vi "get RawTest filename.vi"(10 "Device Name":string, 11 "Wafer Name":string) -> (0 "current time":timestamp, 3 "FileName":string)   [LabVIEW 2012]
uses:
  <vilib>/Utility/miscctls.llb/LVDateTimeRec.ctl
panel:
  out "date/time string":string
  out "date time rec":T1
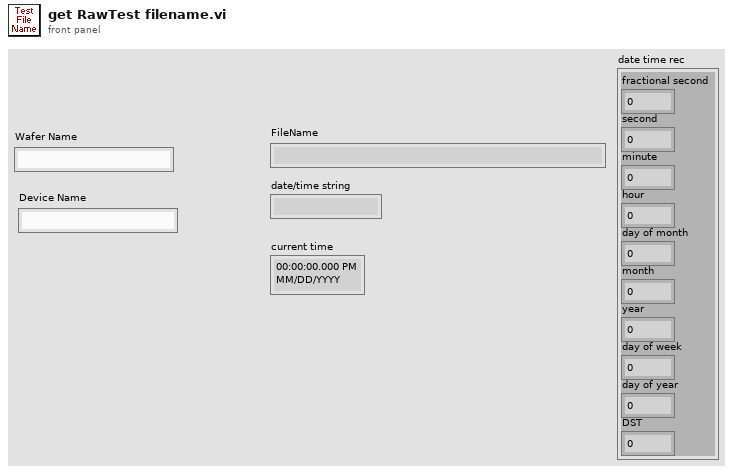
[diagram p1: front panel]
types:
  T1 = typedef "LVDateTimeRec.ctl" = cluster{"fractional second":dbl, "second":i32, "minute":i32, "hour":i32, "day of month":i32, "month":i32, "year":i32, "day of week":i32, "day of year":i32, "DST":i32}
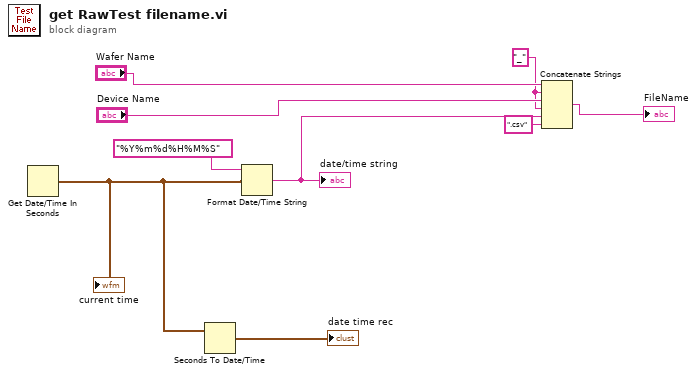
[diagram p0: block diagram]
diagram:
  w7 = "_" ("string")
  n1 = Get Date/Time In Seconds() -> (seconds since 1Jan1904=w4:timestamp)
  "current time" <- w4
  n2 = Seconds To Date/Time(time stamp (now)=w4) -> (date time rec=→"date time rec":T1)  [unwired: 1 in]
  n3 = Format Date/Time String(time format string (%c)="%Y%m%d%H%M%S", seconds (now)=w4) -> (date/time string=w2:string)  [unwired: 1 in]
  "date/time string" <- w2
  n4 = Concatenate Strings("Wafer Name", w7, "Device Name", w7, w2, ".csv" ("string")) -> (→"FileName":string)
